vi "4 графика.vi"() -> ()   [LabVIEW 2021]
panel:
  out "XY Graph":cluster{i32[], dbl[]}(graph)
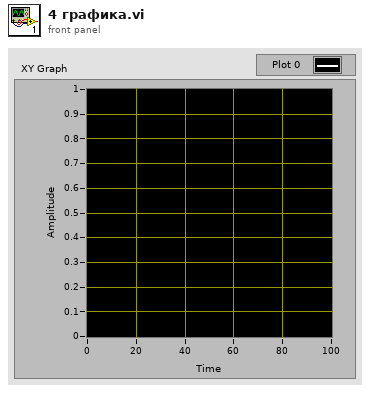
[diagram p1: front panel]
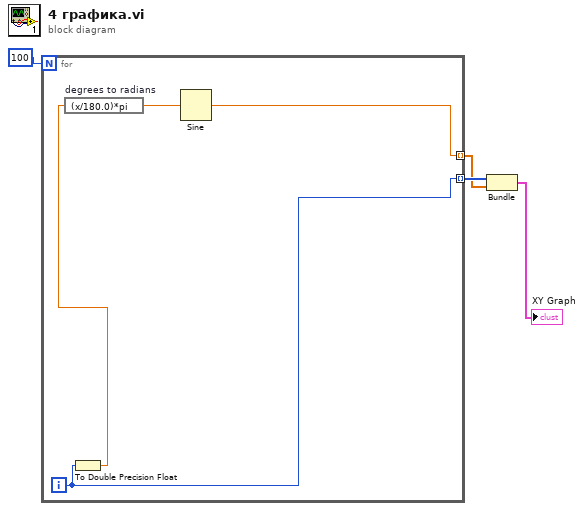
[diagram p0: block diagram]
diagram:
  n1 = for {
    N: 100 -> [_]
    tunnel: [w6] -> w3 mode=indexing
    tunnel: [w5] -> w2 mode=indexing
    i -> [w6]
    n2 = To Double Precision Float(number=w6) -> (double precision float=w7:dbl)
    n3 = expression code="(x/180.0)*pi" "degrees to radians"(w7) -> (w8:dbl)
    n4 = Sine(x=w8) -> (sin(x)=w5:dbl)
  }
  n5 = Bundle(w3, w2) -> (→"XY Graph":cluster{i32[], dbl[]})  [unwired: 1 in]
